vi "to_array.vi"(8 "error in (no error)":errorcluster, 11 "List in":refnum<class "DoublyLinkedList.lvclass">) -> (0 "error out":errorcluster, 2 "data":dbl[](array[numeric]), 3 "List out":refnum<class "DoublyLinkedList.lvclass">)   [LabVIEW 2021, in "DoublyLinkedList.lvclass"]
uses:
  DoublyLinkedList.lvclass
  DoublyLinkedList.lvclass/DoublyLinkedList.ctl
  DoublyNodeRef/DoublyNodeRef.lvclass
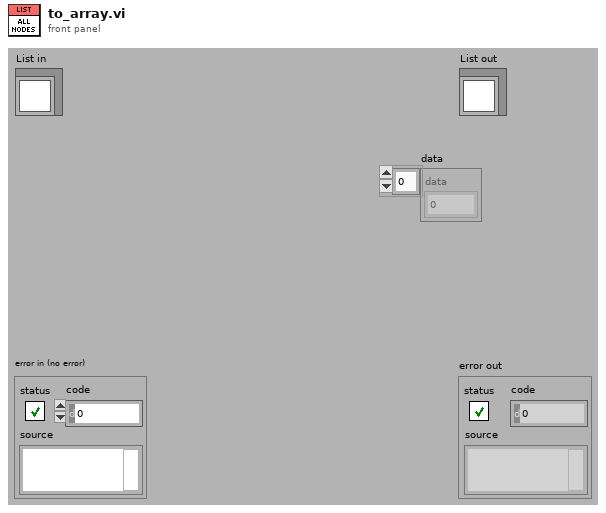
[diagram p1: front panel]
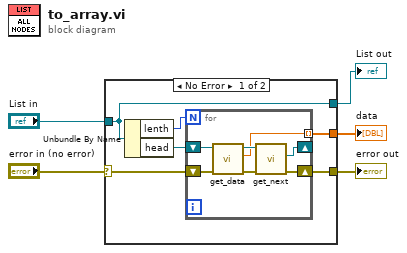
[diagram p0: block diagram]
diagram:
  n1 = case shown="No Error" "error in (no error)" {
    selector: "error in (no error)" -> [w8 w20]
    tunnel: [w11 w20] -> w4
    tunnel: [w6 w19] -> w2
    tunnel: "List in" -> [w6 w19]
    tunnel: [w7 _] -> w1
    frame No Error {
      n2 = Unbundle By Name(w6) -> ("lenth"=w10:u32, "head"=w9:refnum<class "DoublyNodeRef.lvclass">)
      n3 = for {
        N: w10 -> [_]
        shift-right: [w12] -> _
        shift-left: w9 -> [w18]
        shift-right: [w14] -> w11
        shift-left: w8 -> [w17]
        tunnel: [w13] -> w7 mode=indexing
        n4 = call-dynamic "get_data.vi"("error in (no error)"=w17, "DoublyNodeRef in"=w18) -> ("error out"=w15:errorcluster, "data"=w13:dbl, "DoublyNodeRef out"=w16:refnum<class "DoublyNodeRef.lvclass">)  [unwired: 7 in]
        n5 = call-dynamic "get_next.vi"("error in (no error)"=w15, "DoublyNodeRef in"=w16) -> ("error out"=w14:errorcluster, "next"=w12:refnum<class "DoublyNodeRef.lvclass">)  [unwired: 6 in, 2 out]
      }
    }
    frame Error {
    }
  }
  "error out" <- w4
  "List out" <- w2
  "data" <- w1
